vi "testBundleVCluster(Case 13415).vi"() -> ()   [LabVIEW 2011, in "EasyXML_XML_Subset_Source_Tests.lvclass"]
uses:
  EasyXML_XML_Subset_Source_Tests.lvclass
  <vilib>/addons/_JKI Toolkits/VI Tester/TestCase.llb/TestCase.lvclass
panel:
  out "error out":errorcluster
  in  "error in (no error)":errorcluster
  out "EasyXML_XML_Subset_Source_Tests.lvclass":refnum<class "EasyXML_XML_Subset_Source_Tests.lvclass">
  in  "EasyXML_XML_Subset_Source_Tests.lvclass":refnum<class "EasyXML_XML_Subset_Source_Tests.lvclass">
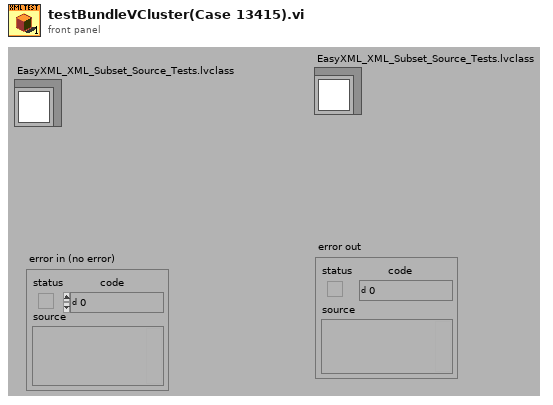
[diagram p1: front panel]
types:
  T1 = cluster{"#attributes":cluster{"VCOSEL":i8, "VCOBND":i8}, "Min_Frequency":dbl, "Max_Frequency":dbl, "Raw_Data":cluster{"VCTRL (V)":dbl[], "Frequency_MHz":dbl[]}}
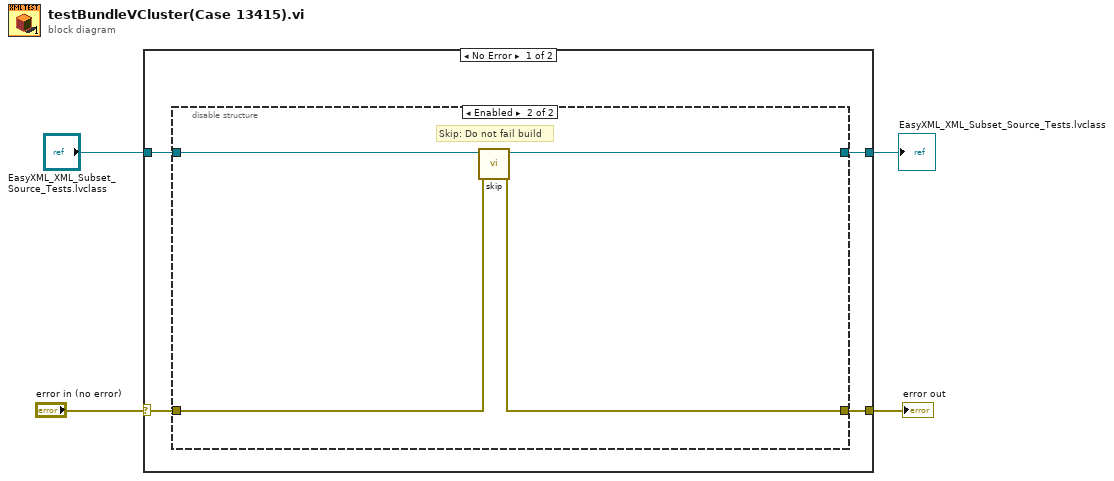
[diagram p0: block diagram]
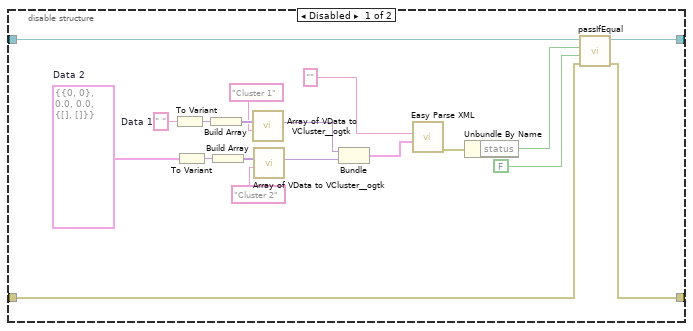
[diagram p2: hidden frame]
diagram:
  n1 = case shown="No Error" "error in (no error)" {
    selector: "error in (no error)" -> [w6 w33]
    tunnel: [w5 w33] -> w3
    tunnel: "EasyXML_XML_Subset_Source_Tests.lvclass" -> [w8 w32]
    tunnel: [w7 w32] -> w1
    frame No Error {
      n2 = disable-structure shown="Enabled" {
        disable-tunnel: w8 -> [w27 w31]
        disable-tunnel: [w26 w30] -> w7
        disable-tunnel: w6 -> [w23 w28]
        disable-tunnel: [w22 w29] -> w5
        frame Disabled {
          w15 = " "  # Data 1
          w21 = T1 {"#attributes"={"VCOSEL"=0, "VCOBND"=0}, "Min_Frequency"=0.0, "Max_Frequency"=0.0, "Raw_Data"={"VCTRL (V)"=[], "Frequency_MHz"=[]}}  # Data 2
          n3 = To Variant(anything=w15) -> (Variant=w18:variant)
          n4 = To Variant(anything=w21) -> (Variant=w20:variant)
          n5 = Build Array(w18) -> (w17:variant[])
          n6 = Build Array(w20) -> (w19:variant[])
          n7 = call <userlib>:"Array of VData to VCluster__ogtk.vi"("Cluster Name"="Cluster 1", "Array"=w17) -> ("VCluster"=w10:variant)  [unwired: 8 in, 1 out]
          n8 = call <userlib>:"Array of VData to VCluster__ogtk.vi"("Cluster Name"="Cluster 2", "Array"=w19) -> ("VCluster"=w9:variant)  [unwired: 8 in, 1 out]
          n9 = Bundle("VCluster"=w10, "VCluster"=w9) -> (w13:cluster{"VCluster":variant, "VCluster":variant})  [unwired: 1 in]
          n10 = call "Easy Parse XML.vi"("LabVIEW Data (Type)"=w13, "XML String"="") -> ("error out"=w11:errorcluster)  [unwired: 8 in, 1 out]
          n11 = Unbundle By Name(w11) -> ("status"=w25:bool)
          n12 = call-dynamic "passIfEqual.vi"("error in (no error)"=w23, "y"=FALSE ("status"), "x"=w25, "TestCase in"=w27) -> ("error out"=w22:errorcluster, "TestCase out"=w26:refnum<class "EasyXML_XML_Subset_Source_Tests.lvclass">)  [unwired: 6 in]
        }
        frame Enabled {
          # "Skip: Do not fail build"
          n13 = call <vilib>:"skip.vi"("error in (no error)"=w28, "TestCase in"=w31) -> ("error out"=w29:errorcluster, "TestCase out"=w30:refnum<class "EasyXML_XML_Subset_Source_Tests.lvclass">)  [unwired: 8 in]
        }
      }
    }
    frame Error {
    }
  }
  "EasyXML_XML_Subset_Source_Tests.lvclass" <- w1
  "error out" <- w3
